vi "testSendServerNotification.vi"(8 "error in (no error)":errorcluster) -> (0 "error out":errorcluster)   [LabVIEW 2018]
doc: "Test the sendServerNotification.vi."
uses:
  src/TcpServerBase/TcpServerBase.lvclass
  src/TcpServerBase/TcpServerBase.lvclass/TcpServerBase.ctl
  <vilib>/addons/_JKI Toolkits/Caraya/classes/Assert/Assert Equal Type_Variant.vi
  <vilib>/addons/_JKI Toolkits/Caraya/classes/Test/Test.lvclass
  <vilib>/addons/_JKI Toolkits/Caraya/classes/Assert/Assert.lvclass
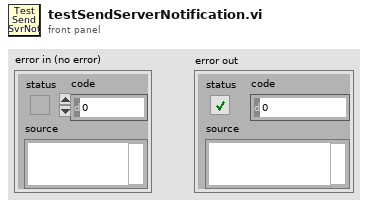
[diagram p1: front panel]
types:
  T1 = cluster{"connectionStatus":bool, "errorSource":string}
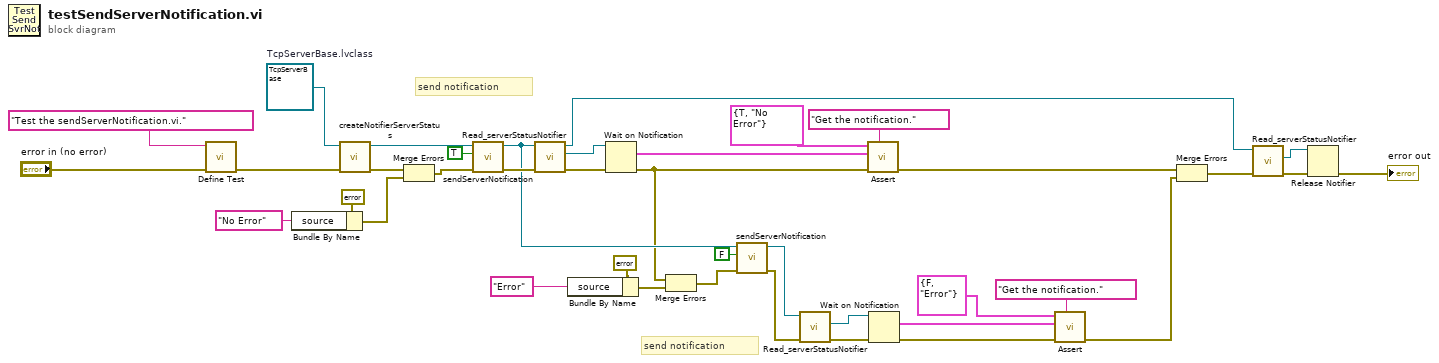
[diagram p0: block diagram]
diagram:
  w36 = refnum<class "TcpServerBase.lvclass"> refnum  # TcpServerBase.lvclass
  # "send notification"
  # "send notification"
  n1 = call <vilib>:"Define Test.vi"("error in (no error)"="error in (no error)", "Label (VI Title)"="Test the sendServerNotification.vi.") -> ("error out"=w35:errorcluster)  [unwired: 9 in]
  n2 = Bundle By Name(cluster=errorcluster {"status"=FALSE, "code"=0, "source"=""} ("error in (no error)"), "source"="No Error") -> (w25:errorcluster)
  n3 = call "createNotifierServerStatus.vi"("error in (no error)"=w35, "tcpServerBase in"=w36) -> ("error out"=w24:errorcluster, "tcpServerBase out"=w34:refnum<class "TcpServerBase.lvclass">)  [unwired: 8 in]
  n4 = Merge Errors(w24, w25) -> (w26:errorcluster)
  n5 = call "sendServerNotification.vi"("error in (no error)"=w26, "connectionStatus"=TRUE ("serverStatus"), "TcpServerBase in"=w34) -> ("error out"=w19:errorcluster, "TcpServerBase out"=w9:refnum<class "TcpServerBase.lvclass">)  [unwired: 7 in]
  n6 = call "Read_serverStatusNotifier.vi"("error in (no error)"=w19, "TcpServerBase in"=w9) -> ("error out"=w32:errorcluster, "serverStatusNotifier"=w31:refnum<notifier>, "TcpServerBase out"=w1:refnum<class "TcpServerBase.lvclass">)  [unwired: 7 in]
  n7 = Bundle By Name(cluster=errorcluster {"status"=FALSE, "code"=0, "source"=""} ("error in (no error)"), "source"="Error") -> (w18:errorcluster)
  n8 = Wait on Notification(notifier=w31, error in (no error)=w32) -> (notification=w27:T1, error out=w8:errorcluster)  [unwired: 2 in, 2 out]
  n9 = Merge Errors(w8, w18) -> (w20:errorcluster)
  n10 = call "sendServerNotification.vi"("error in (no error)"=w20, "connectionStatus"=FALSE ("serverStatus"), "TcpServerBase in"=w9) -> ("error out"=w10:errorcluster, "TcpServerBase out"=w11:refnum<class "TcpServerBase.lvclass">)  [unwired: 7 in]
  n11 = call "Read_serverStatusNotifier.vi"("error in (no error)"=w10, "TcpServerBase in"=w11) -> ("error out"=w13:errorcluster, "serverStatusNotifier"=w14:refnum<notifier>)  [unwired: 7 in, 1 out]
  n12 = call-poly <vilib>:"Assert.vi"("Label"="Get the notification.", "error in (no error)"=w8, "Y"=w27, "X"=T1 {"connectionStatus"=TRUE, "errorSource"="No Error"} ("notification")) -> ("error out"=w7:errorcluster)  [unwired: 7 in]
  n13 = Wait on Notification(notifier=w14, error in (no error)=w13) -> (notification=w17:T1, error out=w15:errorcluster)  [unwired: 2 in, 2 out]
  n14 = call-poly <vilib>:"Assert.vi"("Label"="Get the notification.", "error in (no error)"=w15, "Y"=w17, "X"=T1 {"connectionStatus"=FALSE, "errorSource"="Error"} ("notification")) -> ("error out"=w6:errorcluster)  [unwired: 7 in]
  n15 = Merge Errors(w7, w6) -> (w5:errorcluster)
  n16 = call "Read_serverStatusNotifier.vi"("error in (no error)"=w5, "TcpServerBase in"=w1) -> ("error out"=w4:errorcluster, "serverStatusNotifier"=w2:refnum<notifier>)  [unwired: 7 in, 1 out]
  n17 = Release Notifier(notifier=w2, error in (no error)=w4) -> (error out=→"error out":errorcluster)  [unwired: 1 in, 2 out]
